vi "Update Palette with Ramp.vi"(6 "Control Ref Queue":T1, 8 "error in (no error)":errorcluster, 11 "3D Plot.lvclass in":refnum<class "3D Plot.lvclass">) -> (0 "error out":errorcluster, 1 "Ignore the size change?":bool, 3 "3D Plot.lvclass out":refnum<class "3D Plot.lvclass">)   [LabVIEW 2017, in "3D Plot.lvclass"]
uses:
  <vilib>/Math Plots/3D Math Plots/3D Plot/3D Plot/3D Plot.lvclass
  <vilib>/Math Plots/3D Math Plots/3D Plot/Action String/3DMathPlot Ctrl Act Queue.ctl
  <vilib>/Math Plots/3D Math Plots/3D Plot/Action String/3DMathPlot Ctrl Act Cluster.ctl
  <vilib>/Math Plots/3D Math Plots/3D Plot/Action String/3DMathPlot State Class.ctl
  <vilib>/Math Plots/3D Math Plots/3D Plot/3D Plot/3D Plot.lvclass/3D Plot.ctl
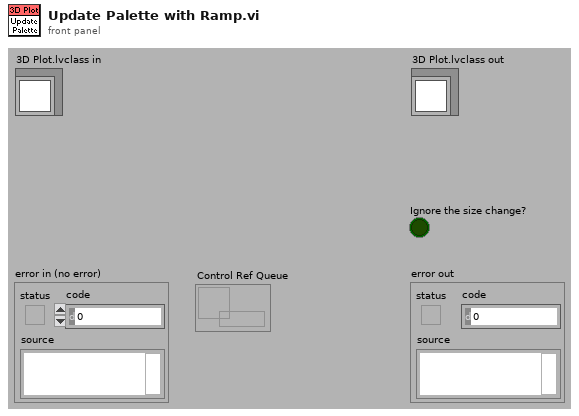
[diagram p1: front panel]
types:
  T1 = typedef "3DMathPlot Ctrl Act Queue.ctl" = refnum<queue>
  T2 = typedef "3DMathPlot Ctrl Act Cluster.ctl" = cluster{"3D Picture Control":refnum<vi>, "Render Window Refnum":refnum<vi>, "XY Graph":refnum<vi>, "Intensity Graph":refnum<vi>, "Color Legend Palette":refnum<vi>, "Projection Palette":refnum<vi>, "XControl  Ref":refnum<vi>, "Facade Ref":refnum<vi>, "Export Image Ref":refnum<vi>, "Clear Data Flag":bool, "Display State Change Class":T3}
  T3 = typedef "3DMathPlot State Class.ctl" = enum16{"Update All Objects (Undo)", "Update Light Object Only", "Update Axis Object Only", "Update Plot Object Only", "Update Cursor Object Only", "Update Axis Plot Cursor Objects", "No Update"}
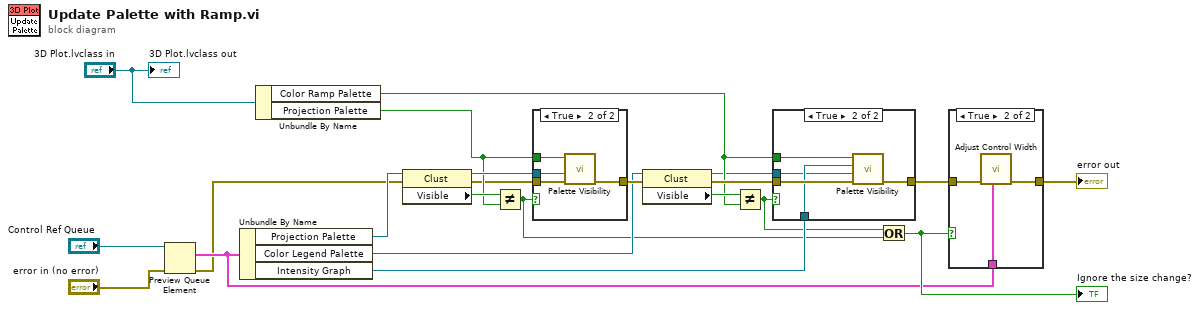
[diagram p0: block diagram]
diagram:
  n1 = Preview Queue Element(queue="Control Ref Queue", error in (no error)="error in (no error)") -> (element=w2:T2, error out=w1:errorcluster)  [unwired: 3 out]
  n2 = Unbundle By Name(w2) -> ("Projection Palette"=w16:refnum<vi>, "Color Legend Palette"=w9:refnum<vi>, "Intensity Graph"=w5:refnum<vi>)
  n3 = Unbundle By Name("3D Plot.lvclass in") -> ("Color Ramp Palette"=w7:bool, "Projection Palette"=w13:bool)
  n4 = property class="Clust"(reference=w16, error in=w1) -> (reference out=w15:refnum<vi>, error out=w12:errorcluster, "Visible"=w14:bool)
  n5 = Not Equal?(x=w14, y=w13) -> (x != y?=w4:bool)
  n6 = case shown="True" w4 {
    tunnel: [w23 w27] -> w11
    tunnel: w12 -> [w23 w26]
    tunnel: w15 -> [_ w25]
    tunnel: w13 -> [_ w24]
    frame False {
    }
    frame True {
      n7 = call <vilib>:"Palette Visibility.vi"("error in (no error)"=w26, "Clust Refnum"=w25, "Visible?"=w24) -> ("error out"=w27:errorcluster)  [unwired: 1 in, 7 out]
    }
  }
  n8 = property class="Clust"(reference=w9, error in=w11) -> (reference out=w6:refnum<vi>, error out=w10:errorcluster, "Visible"=w8:bool)
  n9 = Not Equal?(x=w8, y=w7) -> (x != y?=w3:bool)
  n10 = case shown="True" w3 {
    tunnel: w7 -> [_ w33]
    tunnel: w10 -> [w28 w32]
    tunnel: w5 -> [_ w31]
    tunnel: w6 -> [_ w30]
    tunnel: [w28 w29] -> w17
    frame False {
    }
    frame True {
      n11 = call <vilib>:"Palette Visibility.vi"("error in (no error)"=w32, "Clust Refnum"=w30, "IntGraph Refnum"=w31, "Visible?"=w33) -> ("error out"=w29:errorcluster)  [unwired: 7 out]
    }
  }
  n12 = Or(x=w3, y=w4) -> (x .or. y?=w20:bool)
  "Ignore the size change?" <- w20
  n13 = case shown="True" w20 {
    tunnel: w17 -> [w34 w37]
    tunnel: [w34 w36] -> w21
    tunnel: w2 -> [_ w35]
    frame False {
    }
    frame True {
      n14 = call <vilib>:"Adjust Control Width.vi"("Control Ref Cluster"=w35, "error in (no error)"=w37) -> ("error out"=w36:errorcluster)  [unwired: 9 out]
    }
  }
  "error out" <- w21
  "3D Plot.lvclass out" <- "3D Plot.lvclass in"
